vi "UI - Initialize IO Variables.vi"(8 "error in (no error)":errorcluster, 11 "Controller Address":string) -> (0 "error out":errorcluster, 3 "IO References":T1)   [LabVIEW 2014]
uses:
  Controls/IO References.ctl
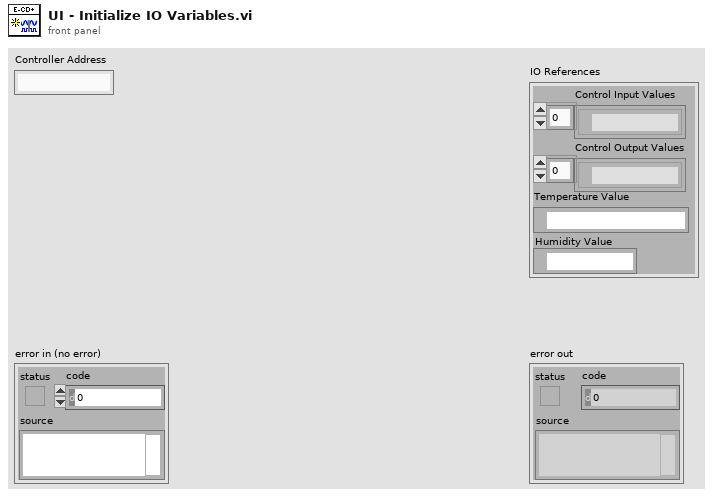
[diagram p1: front panel]
types:
  T1 = typedef "IO References.ctl" = cluster{"Control Input Values":refnum<k21>[], "Control Output Values":refnum<k21>[], "Temperature Value":refnum<k21>, "Humidity Value":refnum<k21>}
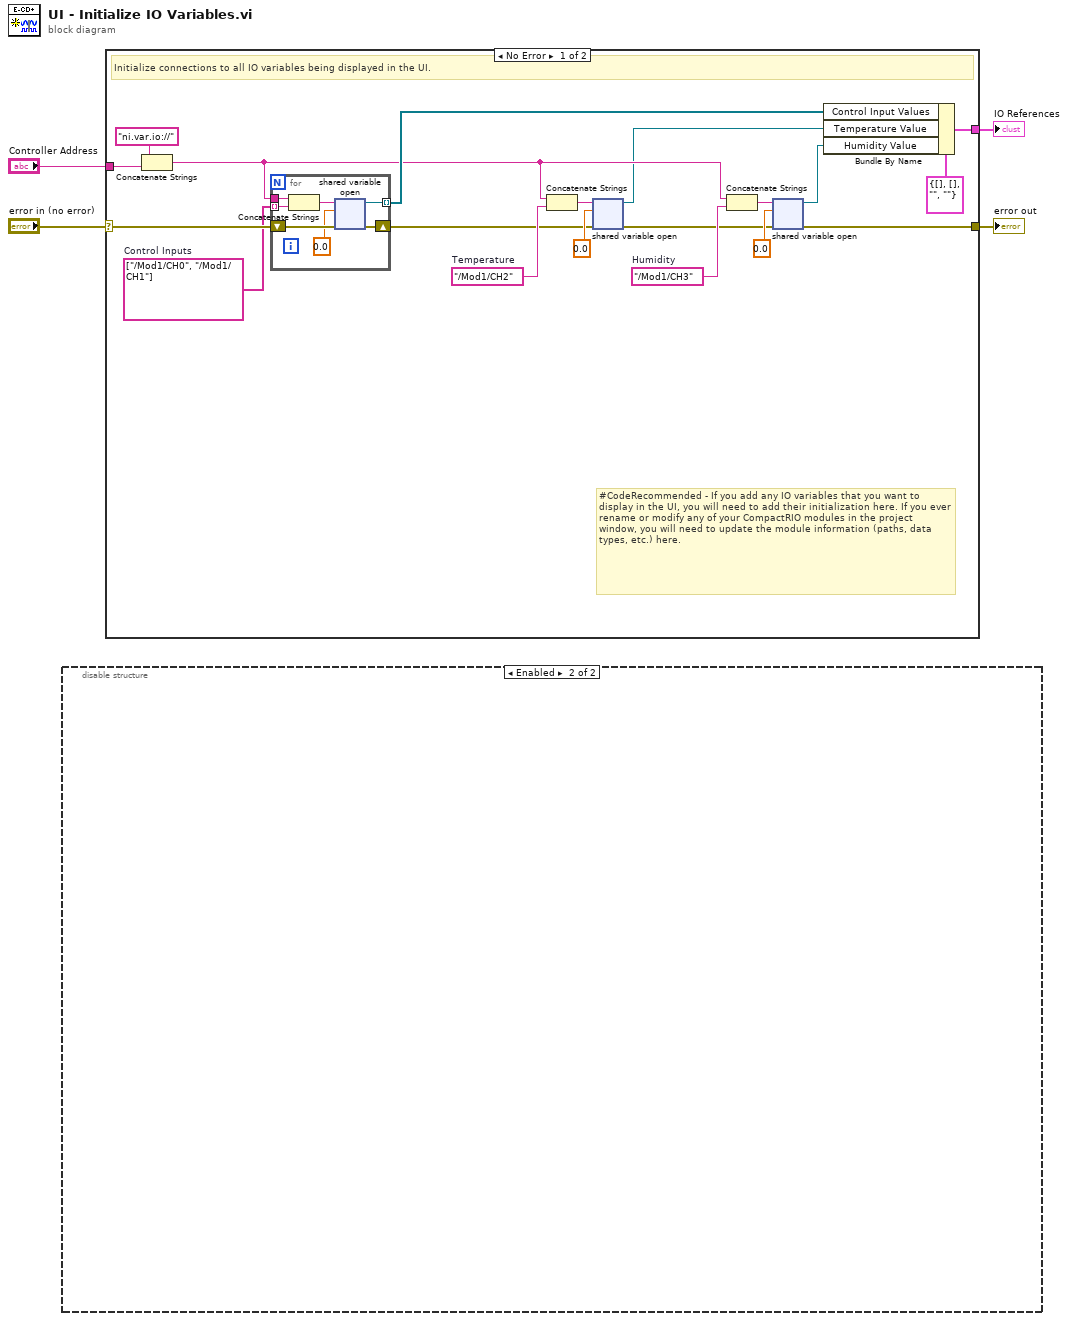
[diagram p0: block diagram]
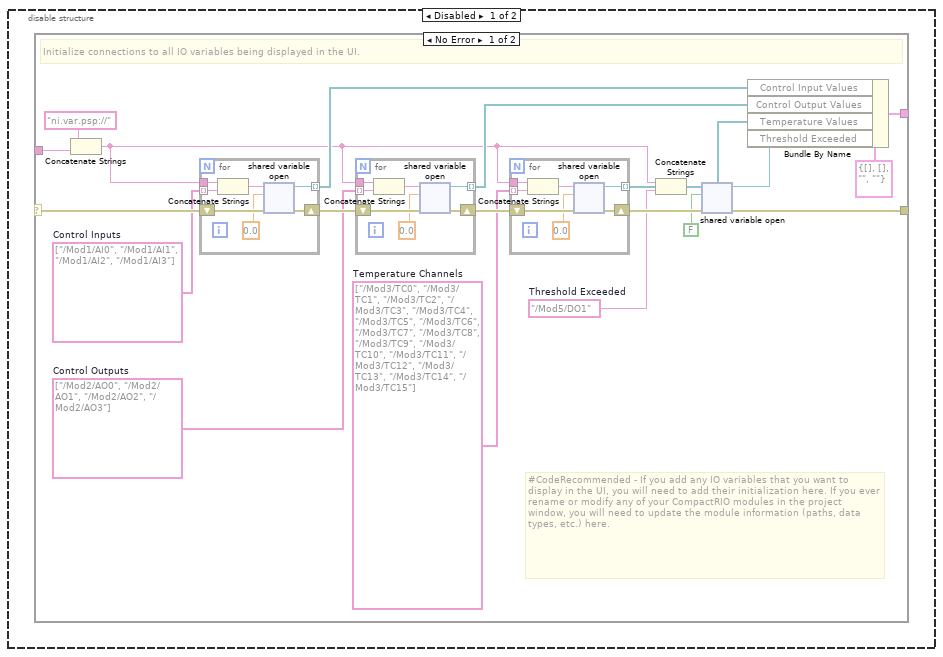
[diagram p2: hidden frame]
diagram:
  n1 = disable-structure shown="Enabled" {
    frame Disabled {
      n2 = case shown="No Error" {
        selector: _ -> [w21 w46]
        tunnel: _ -> [w23 _]
        tunnel: [w5 w46] -> _
        tunnel: [w18 _] -> _
        frame No Error {
          w9 = "/Mod5/DO1"  # Threshold Exceeded
          w13 = string[] ["/Mod3/TC0", "/Mod3/TC1", "/Mod3/TC2", "/Mod3/TC3", "/Mod3/TC4", "/Mod3/TC5", "/Mod3/TC6", "/Mod3/TC7", "/Mod3/TC8", "/Mod3/TC9", "/Mod3/TC10", "/Mod3/TC11", "/Mod3/TC12", "/Mod3/TC13", "/Mod3/TC14", "/Mod3/TC15"]  # Temperature Channels
          w16 = string[] ["/Mod2/AO0", "/Mod2/AO1", "/Mod2/AO2", "/Mod2/AO3"]  # Control Outputs
          w20 = string[] ["/Mod1/AI0", "/Mod1/AI1", "/Mod1/AI2", "/Mod1/AI3"]  # Control Inputs
          # "#CodeRecommended - If you add any IO variables that you want to display in the UI, you will need to add their initialization here. If you ever rename or modify any of your CompactRIO modules in the project window, you will need to update the module information (paths, data types, etc.) here."
          # "Initialize connections to all IO variables being displayed in the UI."
          n3 = Concatenate Strings("ni.var.psp://", w23) -> (w11:string)
          n4 = for {
            shift-right: [w44] -> w17
            shift-left: w21 -> [w45]
            tunnel: w11 -> [w41]
            tunnel: w20 -> [w40] mode=indexing
            tunnel: [w39] -> w19 mode=indexing
            n5 = Concatenate Strings(w41, w40) -> (w43:string)
            n6 = shared-variable-open(w43, w45, 0.0) -> (w39:refnum<k21>, w44:errorcluster)  [unwired: 1 in]
          }
          n7 = for {
            shift-right: [w37] -> w14
            shift-left: w17 -> [w38]
            tunnel: w11 -> [w34]
            tunnel: w16 -> [w33] mode=indexing
            tunnel: [w32] -> w15 mode=indexing
            n8 = Concatenate Strings(w34, w33) -> (w36:string)
            n9 = shared-variable-open(w36, w38, 0.0) -> (w32:refnum<k21>, w37:errorcluster)  [unwired: 1 in]
          }
          n10 = for {
            shift-right: [w30] -> w10
            shift-left: w14 -> [w31]
            tunnel: w11 -> [w27]
            tunnel: w13 -> [w26] mode=indexing
            tunnel: [w25] -> w12 mode=indexing
            n11 = Concatenate Strings(w27, w26) -> (w29:string)
            n12 = shared-variable-open(w29, w31, 0.0) -> (w25:refnum<k21>, w30:errorcluster)  [unwired: 1 in]
          }
          n13 = Concatenate Strings(w11, w9) -> (w8:string)
          n14 = shared-variable-open(w8, w10, FALSE) -> (w6:refnum<k21>, w5:errorcluster)  [unwired: 1 in]
          n15 = Bundle By Name(cluster=T1 {"Control Input Values"=[], "Control Output Values"=[], "Temperature Value"="", "Humidity Value"=""} ("IO References"), "Control Input Values"=w19, "Control Output Values"=w15, "Temperature Values"=w12, "Threshold Exceeded"=w6) -> (w18:T1)
        }
        frame Error {
          # "Error"
        }
      }
    }
    frame Enabled {
    }
  }
  n16 = case shown="No Error" "error in (no error)" {
    selector: "error in (no error)" -> [w62 w73]
    tunnel: "Controller Address" -> [w64 _]
    tunnel: [w56 w73] -> w2
    tunnel: [w59 _] -> w1
    frame No Error {
      w52 = "/Mod1/CH2"  # Temperature
      w58 = "/Mod1/CH3"  # Humidity
      w61 = string[] ["/Mod1/CH0", "/Mod1/CH1"]  # Control Inputs
      # "#CodeRecommended - If you add any IO variables that you want to display in the UI, you will need to add their initialization here. If you ever rename or modify any of your CompactRIO modules in the project window, you will need to update the module information (paths, data types, etc.) here."
      # "Initialize connections to all IO variables being displayed in the UI."
      n17 = Concatenate Strings("ni.var.io://", w64) -> (w51:string)
      n18 = for {
        shift-right: [w71] -> w50
        shift-left: w62 -> [w72]
        tunnel: w51 -> [w68]
        tunnel: w61 -> [w67] mode=indexing
        tunnel: [w66] -> w60 mode=indexing
        n19 = Concatenate Strings(w68, w67) -> (w70:string)
        n20 = shared-variable-open(w70, w72, 0.0) -> (w66:refnum<k21>, w71:errorcluster)  [unwired: 1 in]
      }
      n21 = Concatenate Strings(w51, w52) -> (w53:string)
      n22 = shared-variable-open(w53, w50, 0.0) -> (w48:refnum<k21>, w49:errorcluster)  [unwired: 1 in]
      n23 = Concatenate Strings(w51, w58) -> (w57:string)
      n24 = shared-variable-open(w57, w49, 0.0) -> (w47:refnum<k21>, w56:errorcluster)  [unwired: 1 in]
      n25 = Bundle By Name(cluster=T1 {"Control Input Values"=[], "Control Output Values"=[], "Temperature Value"="", "Humidity Value"=""} ("IO References"), "Control Input Values"=w60, "Temperature Value"=w48, "Humidity Value"=w47) -> (w59:T1)
    }
    frame Error {
      # "Error"
    }
  }
  "error out" <- w2
  "IO References" <- w1
